vi "Plot3.vi"(8 "error constant":errorcluster, 9 "Reset":bool caption="Checkbox", 11 "Array 2":waveform(dbl)[](array[waveform])) -> (0 "error constant 2":errorcluster, 1 "DoneReset":bool, 3 "Waveform Chart":waveform(dbl)[](graph))   [LabVIEW 2023]
panel:
  out "size(s)":i32
  in  "Time Length s":dbl=5.0 min=1e-11 max=1000000000000.0
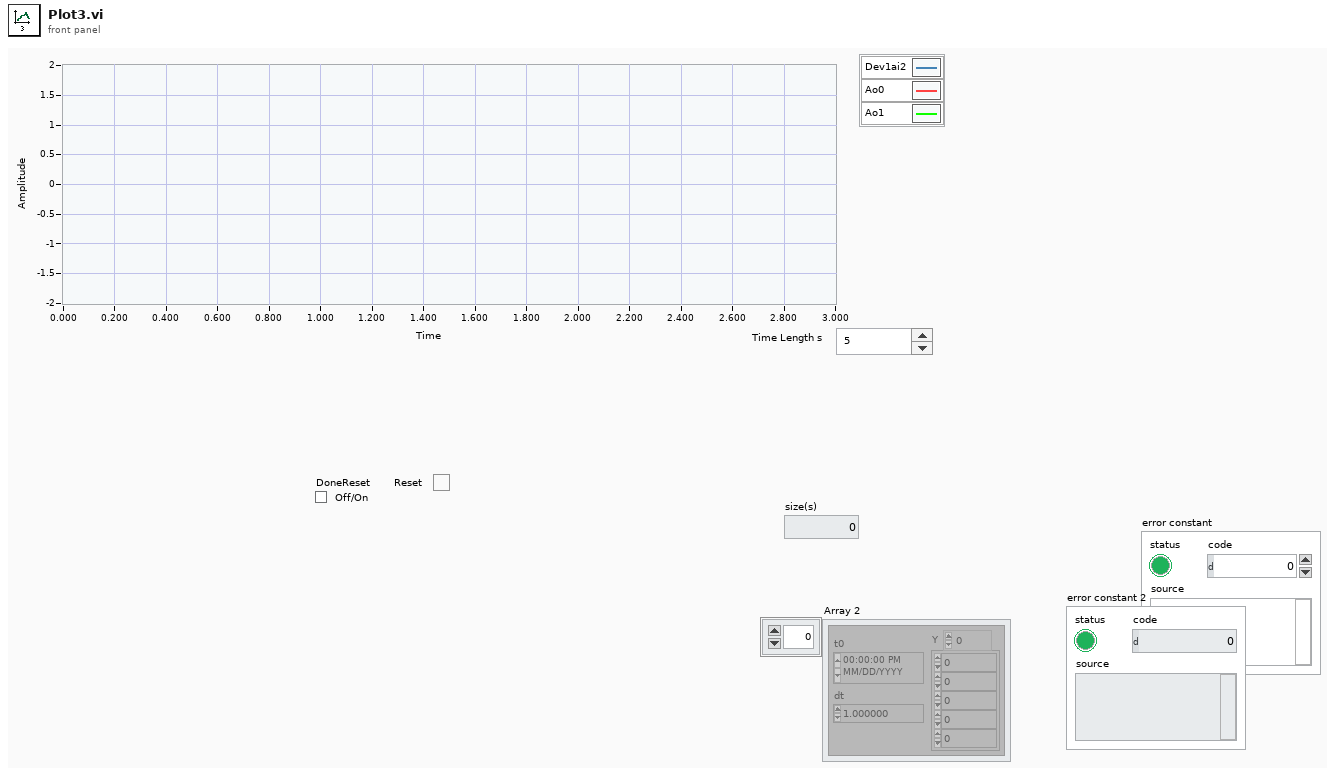
[diagram p1: front panel]
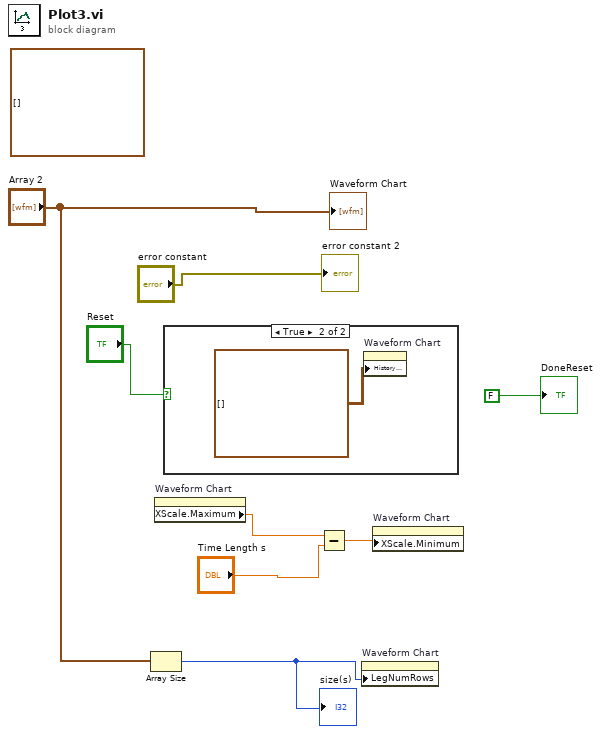
[diagram p0: block diagram]
diagram:
  (unwired) waveform(dbl)[] []
  n1 = Array Size(array="Array 2") -> (size(s)=w2:i32)
  "size(s)" <- w2
  n2 = property on="Waveform Chart" class="WFChart (strict)"() -> ("XScale.Maximum"=w4:dbl)  [unwired: 2 in, 2 out]
  n3 = case shown="True" "Reset" {
    frame False {
    }
    frame True {
      n4 = property on="Waveform Chart" class="WFChart (strict)"("History Data"=waveform(dbl)[][] []) -> ()  [unwired: 2 in, 2 out]
    }
  }
  n5 = Subtract(x=w4, y="Time Length s") -> (x-y=w5:dbl)
  n6 = property on="Waveform Chart" class="WFChart (strict)"("LegNumRows"=w2) -> ()  [unwired: 2 in, 2 out]
  n7 = property on="Waveform Chart" class="WFChart (strict)"("XScale.Minimum"=w5) -> ()  [unwired: 2 in, 2 out]
  "Waveform Chart" <- "Array 2"
  "error constant 2" <- "error constant"
  "DoneReset" <- FALSE
